vi "Write Message Queue.vi"(8 "error in (no error)":errorcluster, 10 "Message Queue":T1, 11 "Map Tree Queue Messenger in":refnum<class "Map Tree Queue Messenger.lvclass">) -> (0 "error out":errorcluster, 3 "Map Tree Queue Messenger out":refnum<class "Map Tree Queue Messenger.lvclass">)   [LabVIEW 2024, in "Map Tree Queue Messenger.lvclass"]
uses:
  Map Tree Queue Messenger.lvclass
  Simple Tree Queue Messenger/Type Def/Message Queue.ctl
  Ancestor Class/Message/Message.lvclass
  Map Tree Queue Messenger.lvclass/Map Tree Queue Messenger.ctl
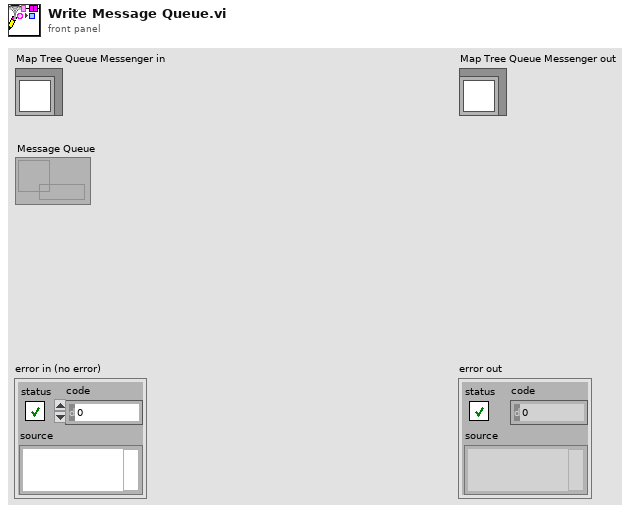
[diagram p1: front panel]
types:
  T1 = typedef "Message Queue.ctl" = refnum<queue>
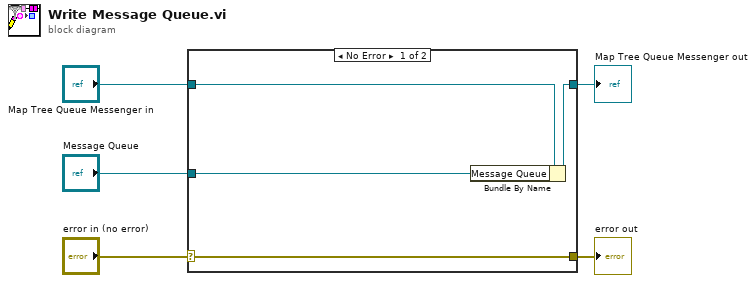
[diagram p0: block diagram]
diagram:
  n1 = case shown="No Error" "error in (no error)" {
    selector: "error in (no error)" -> [w9 w10]
    tunnel: [w9 w10] -> w4
    tunnel: [w7 w11] -> w2
    tunnel: "Map Tree Queue Messenger in" -> [w8 w11]
    tunnel: "Message Queue" -> [w6 _]
    frame No Error {
      n2 = Bundle By Name(cluster=w8, "Message Queue"=w6) -> (w7:refnum<class "Map Tree Queue Messenger.lvclass">)
    }
    frame Error {
    }
  }
  "error out" <- w4
  "Map Tree Queue Messenger out" <- w2
